vi "Downconvert complex waveform.vi"(6 "Enable Sw DDC":bool=TRUE, 8 "error in (no error)":errorcluster, 9 "passband bandwidth (Hz)":dbl, 10 "carrier frequency (Hz)":dbl, 11 "CDB Wfm in":waveform(cdb)) -> (0 "error out":errorcluster, 3 "output waveform out":waveform(cdb))   [LabVIEW 2015, in "Monitoring_receiver.lvlib"]
uses:
  Monitoring_receiver.lvlib
  <vilib>/measure/NI_MAPro.lvlib
  <vilib>/measure/maspectr.llb/FFT Power Spectrum and PSD for 1 Chan (CDB).vi
panel:
  out "Power Spectrum / PSD":cluster{"f0":dbl, "df":dbl, "magnitude":dbl[]}(graph)
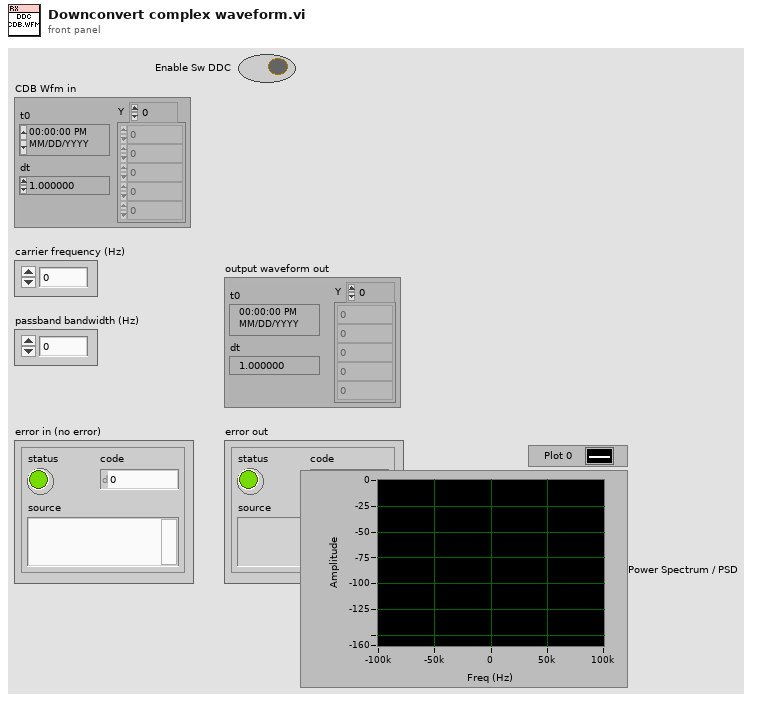
[diagram p1: front panel]
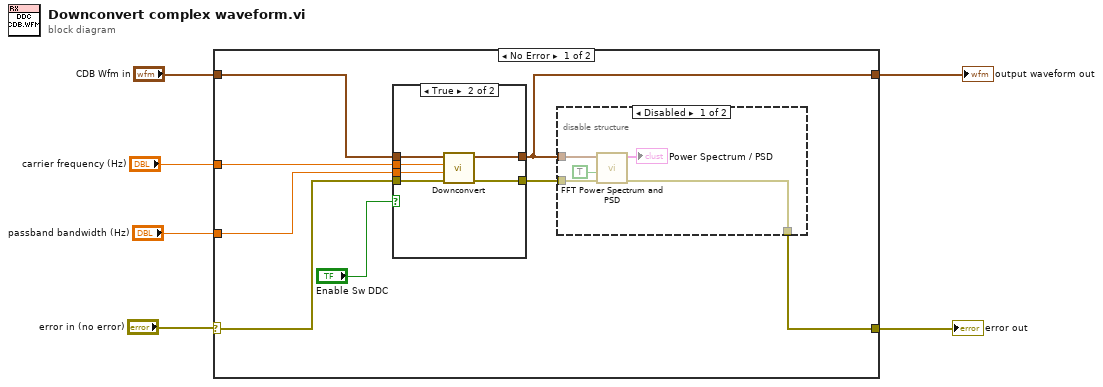
[diagram p0: block diagram]
diagram:
  n1 = case shown="No Error" "error in (no error)" {
    selector: "error in (no error)" -> [w12 w30]
    tunnel: "carrier frequency (Hz)" -> [w14 _]
    tunnel: "passband bandwidth (Hz)" -> [w13 _]
    tunnel: [w7 w30] -> w3
    tunnel: "CDB Wfm in" -> [w11 w29]
    tunnel: [w9 w29] -> w6
    frame No Error {
      n2 = case shown="True" "Enable Sw DDC" {
        tunnel: w14 -> [_ w28]
        tunnel: w13 -> [_ w27]
        tunnel: [w21 w26] -> w8
        tunnel: w12 -> [w21 w25]
        tunnel: w11 -> [w22 w24]
        tunnel: [w22 w23] -> w9
        frame False {
        }
        frame True {
          n3 = call "Downconvert.vi"("error in (no error)"=w25, "passband bandwidth (Hz)"=w27, "carrier frequency (Hz)"=w28, "CDB Wfm in"=w24) -> ("error out"=w26:errorcluster, "CDB Wfm out"=w23:waveform(cdb))  [unwired: 6 in]
        }
      }
      n4 = disable-structure shown="Disabled" {
        disable-tunnel: w9 -> [w17 _]
        disable-tunnel: w8 -> [w16 w20]
        disable-tunnel: [w15 w20] -> w7
        frame Disabled {
          n5 = call-poly <vilib>:"FFT Power Spectrum and PSD.vi"("error in (no error)"=w16, "dB On (F)"=TRUE, "time signal"=w17) -> ("error out"=w15:errorcluster, "Power Spectrum / PSD"=→"Power Spectrum / PSD":cluster{"f0":dbl, "df":dbl, "magnitude":dbl[]})  [unwired: 5 in, 2 out]
        }
        frame Enabled {
        }
      }
    }
    frame Error {
    }
  }
  "output waveform out" <- w6
  "error out" <- w3
